vi "Timing Calculator_v2.vi"(8 "Scan settings array":T1[](array[typedef]) {"J-t Illumination conditions" items=["Light only", "Dark only", "Light then dark", "Dark then light"]; "No. of scan rate steps" min=1.0 step=1.0; "Illumination conditions" items=["Light only", "Dark only", "Light then dark", "Dark then light", "Light then dark then light", "Dark then light then dark"]; "Time Constant (s)" items=["0.01s", "0.03s", "0.1s", "0.3s", "1s", "3s"]; "Only repeat for best pixel" items=["only for best pixel", "for best 2 pixels", "for best 3 pixels", "for best 4 pixels", "for best 5 pixels", "for best 6 pixels", "for best 7 pixels", "for all pixels"]; "No. of repeat scans" min=1.0 step=1.0; "EQE best pixel only" items=["only the best pixel", "the best 2 pixel", "the best 3 pixel", "the best 4 pixel", "the best 5 pixel", "the best 6 pixel", "the best 7 pixel", "all pixels"]; "P dep best pixel only" items=["only the best pixel", "the best 2 pixels", "the best 3 pixels", "the best 4 pixels", "the best 5 pixels", "the best 6 pixels", "the best 7 pixels", "all pixels"]; "Max power best pixel only" items=["only the best pixel", "the best 2 pixels", "the best 3 pixels", "the best 4 pixels", "the best 5 pixels", "the best 6 pixels", "the best 7 pixels", "all pixels"]; "J-t best pixel only" items=["only the best pixel", "the best 2 pixels", "the best 3 pixels", "the best 4 pixels", "the best 5 pixels", "the best 6 pixels", "the best 7 pixels", "all pixels"]; "Integration time" items=["Fast", "Normal", "High Accuracy"]; "Stabilisation mode" items=["V", "I"]; "Measurement delay (ms)" min=10.0}, 11 "Measurement queue":T3(array[cluster]) {"Pixel to measure" items=["All", "1", "2", "3", "4", "5", "6", "7", "8"]}) -> (3 "Experiment time (s)":dbl)   [LabVIEW 2011]
uses:
  TypeDefs/Scan settings.ctl
  TypeDefs/Settings Boolean.ctl
panel:
  out "Step time (s)":dbl
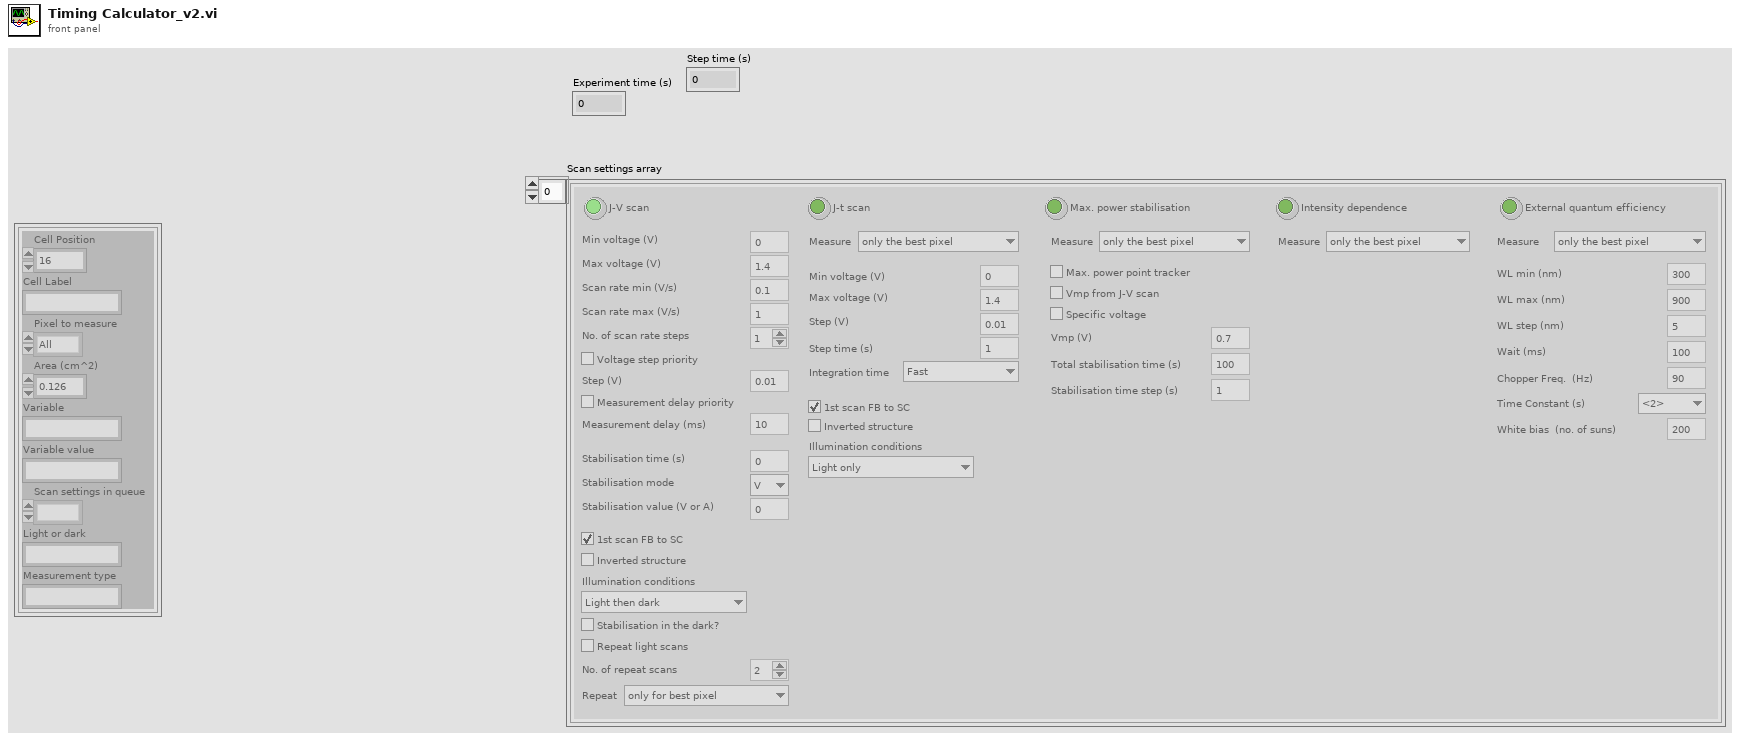
[diagram p1: front panel]
types:
  T1 = typedef "Scan settings.ctl" = cluster{"J-V scan":T2, "J-t scan":bool, "Min voltage (V)":dbl, "Max voltage (V)":dbl, "Step (V)":dbl, "Measurement delay (ms)":dbl, "1st scan FB-SC":bool, "Inverted structure":bool, "Stabilisation time (s)":dbl, "Stabilisation mode":u16, "Stabilisation value (V or A) ":dbl, "Step time (s)":dbl, "Integration time":u16, "Repeat light scans":bool, "Stabilisation in the dark?":bool, "J-t Min (V)":dbl, "J-t Max (V)":dbl, "J-t Step (V)":dbl, "Max. power stabilisation":bool, "J-t 1st scan FB-SC":bool, "J-t Inverted structure":bool, "Max power tracking":bool, "Vmp (V)":dbl, "Total stabilisation time (s)":dbl, "J-t best pixel only":u16, "Max power best pixel only":u16, "Vmp from J-V scan":bool, "Intensity dependence":bool, "P dep best pixel only":u16, "External quantum efficiency":bool, "EQE best pixel only":u16, "WL min (nm)":dbl, "WL max (nm)":dbl, "WL step (nm)":dbl, "Wait (ms)":dbl, "No. of repeat scans":dbl, "Only repeat for best pixel":u16, "Chopper Freq.  (Hz)":dbl, "Time Constant (s)":dbl, "Stabilisation time step (s)":dbl, "Illumination conditions":u16, "Scan rate min (V/s)":dbl, "Scan rate max (V/s)":dbl, "No. of scan rate steps":dbl, "Scan rate voltage step priority":bool, "Scan rate measurement delay priority":bool, "J-t Illumination conditions":u16, "White bias  (no. of suns)":dbl, "Max P stab. Specific voltage":bool}
  T2 = typedef "Settings Boolean.ctl" = bool
  T3 = cluster{"Cell Position":i32, "Cell Label":string, "Pixel to measure":u16, "Area (cm^2)":dbl, "Variable":string, "Variable value":string, "Scan settings in queue":u16, "Light or dark":string, "Measurement type":string}[]
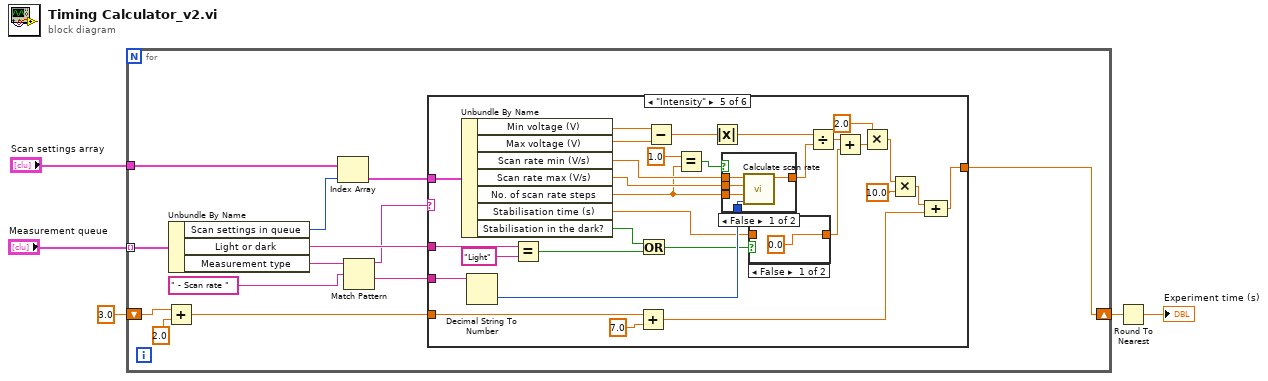
[diagram p0: block diagram]
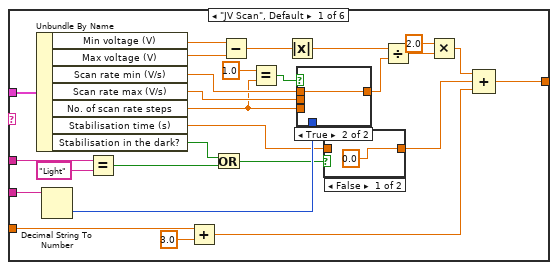
[diagram p2: hidden frame]
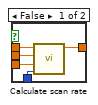
[diagram p4: hidden frame]
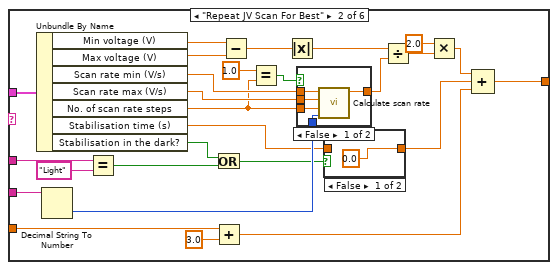
[diagram p5: hidden frame]
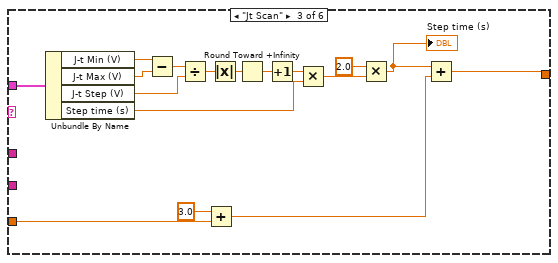
[diagram p8: hidden frame]
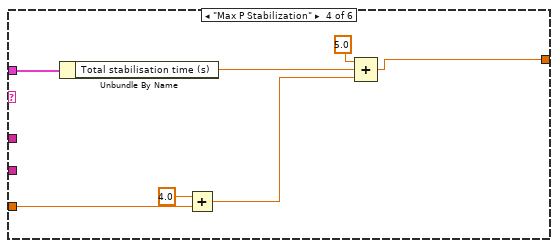
[diagram p9: hidden frame]
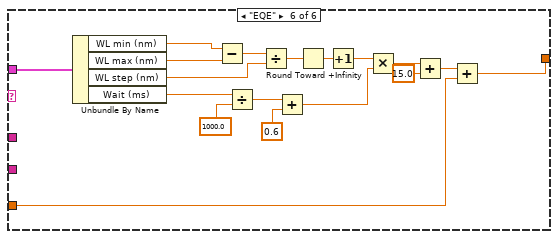
[diagram p12: hidden frame]
diagram:
  n1 = for {
    tunnel: "Measurement queue" -> [w18] mode=indexing
    shift-right: [w6] -> w1
    shift-left: 3.0 -> [w8]
    tunnel: "Scan settings array" -> [w10]
    n2 = Add(x=w8, y=2.0) -> (x+y=w11:dbl)
    n3 = Unbundle By Name(w18) -> ("Scan settings in queue"=w17:u16, "Light or dark"=w12:string, "Measurement type"=w13:string)
    n4 = Index Array(array=w10, index=w17) -> (element=w16:T1)
    n5 = Match Pattern(string=w13, regular expression=" - Scan rate ") -> (before substring=w9:string, after substring=w14:string)  [unwired: 1 in, 2 out]
    n6 = case shown="\"Intensity\"" w9 {
      tunnel: [w43 w78 w97 w109 w126 w151] -> w6
      tunnel: w16 -> [w42 w77 w98 w111 w125 w153]
      tunnel: w14 -> [w40 w75 _ _ w119 _]
      tunnel: w12 -> [w31 w66 _ _ w124 _]
      tunnel: w11 -> [w21 w55 w94 w108 w114 w152]
      frame "JV Scan", Default {
        n7 = Unbundle By Name(w42) -> ("Min voltage (V)"=w45:dbl, "Max voltage (V)"=w44:dbl, "Scan rate min (V/s)"=w37:dbl, "Scan rate max (V/s)"=w38:dbl, "No. of scan rate steps"=w35:dbl, "Stabilisation time (s)"=w29:dbl, "Stabilisation in the dark?"=w28:bool)
        n8 = Decimal String To Number(string=w40) -> (number=w39:i32)  [unwired: 2 in, 1 out]
        n9 = Equal?(x=w31, y="Light") -> (x = y?=w26:bool)
        n10 = Add(x=w21, y=3.0) -> (x+y=w20:dbl)
        n11 = Or(x=w28, y=w26) -> (x .or. y?=w27:bool)
        n12 = Subtract(x=w45, y=w44) -> (x-y=w41:dbl)
        n13 = Equal?(x=1.0 ("y"), y=w35) -> (x = y?=w34:bool)
        n14 = Absolute Value(x=w41) -> (abs(x)=w33:dbl)
        n15 = case shown="True" w34 {
          tunnel: w39 -> [w52 _]
          tunnel: w35 -> [w51 _]
          tunnel: w38 -> [w50 _]
          tunnel: w37 -> [w49 w53]
          tunnel: [w48 w53] -> w32
          frame False {
            n16 = call "Calculate scan rate.vi"("Scan rate number"=w52, "Number of steps"=w51, "Scan rate max (V/s)"=w50, "Scan rate min (V/s)"=w49) -> ("Scan rate"=w48:dbl)  [unwired: 7 in]
          }
          frame True {
          }
        }
        n17 = case shown="False" w27 {
          tunnel: w29 -> [_ w47]
          tunnel: [0.0 ("Stabilisation time (s)") w47] -> w25
          frame False {
          }
          frame True {
          }
        }
        n18 = Divide(x=w33, y=w32) -> (x/y=w24:dbl)
        n19 = Multiply(x=2.0, y=w24) -> (x*y=w22:dbl)
        n20 = Compound Arithmetic op=ADD(w22, w25, w20) -> (w43:dbl)
      }
      frame "Repeat JV Scan For Best" {
        n21 = Unbundle By Name(w77) -> ("Min voltage (V)"=w80:dbl, "Max voltage (V)"=w79:dbl, "Scan rate min (V/s)"=w72:dbl, "Scan rate max (V/s)"=w73:dbl, "No. of scan rate steps"=w70:dbl, "Stabilisation time (s)"=w64:dbl, "Stabilisation in the dark?"=w63:bool)
        n22 = Decimal String To Number(string=w75) -> (number=w74:i32)  [unwired: 2 in, 1 out]
        n23 = Equal?(x=w66, y="Light") -> (x = y?=w61:bool)
        n24 = Or(x=w63, y=w61) -> (x .or. y?=w62:bool)
        n25 = Add(x=w55, y=3.0) -> (x+y=w54:dbl)
        n26 = Subtract(x=w80, y=w79) -> (x-y=w76:dbl)
        n27 = Equal?(x=1.0 ("y"), y=w70) -> (x = y?=w69:bool)
        n28 = Absolute Value(x=w76) -> (abs(x)=w68:dbl)
        n29 = case shown="False" w69 {
          tunnel: w74 -> [w87 _]
          tunnel: w70 -> [w86 _]
          tunnel: w73 -> [w85 _]
          tunnel: w72 -> [w84 w88]
          tunnel: [w83 w88] -> w67
          frame False {
            n30 = call "Calculate scan rate.vi"("Scan rate number"=w87, "Number of steps"=w86, "Scan rate max (V/s)"=w85, "Scan rate min (V/s)"=w84) -> ("Scan rate"=w83:dbl)  [unwired: 7 in]
          }
          frame True {
          }
        }
        n31 = case shown="False" w62 {
          tunnel: w64 -> [_ w82]
          tunnel: [0.0 ("Stabilisation time (s)") w82] -> w60
          frame False {
          }
          frame True {
          }
        }
        n32 = Divide(x=w68, y=w67) -> (x/y=w59:dbl)
        n33 = Multiply(x=2.0, y=w59) -> (x*y=w58:dbl)
        n34 = Compound Arithmetic op=ADD(w58, w60, w54) -> (w78:dbl)
      }
      frame "Jt Scan" {
        n35 = Unbundle By Name(w98) -> ("J-t Min (V)"=w99:dbl, "J-t Max (V)"=w100:dbl, "J-t Step (V)"=w102:dbl, "Step time (s)"=w105:dbl)
        n36 = Subtract(x=w99, y=w100) -> (x-y=w101:dbl)
        n37 = Divide(x=w101, y=w102) -> (x/y=w90:dbl)
        n38 = Add(x=3.0, y=w94) -> (x+y=w93:dbl)
        n39 = Absolute Value(x=w90) -> (abs(x)=w89:dbl)
        n40 = Round Toward +Infinity(x=w89) -> (ceil(x): smallest int >= x=w103:dbl)
        n41 = Increment(x=w103) -> (x+1=w104:dbl)
        n42 = Multiply(x=w104, y=w105) -> (x*y=w96:dbl)
        n43 = Multiply(x=2.0, y=w96) -> (x*y=w91:dbl)
        "Step time (s)" <- w91
        n44 = Add(x=w91, y=w93) -> (x+y=w97:dbl)
      }
      frame "Max P Stabilization" {
        n45 = Unbundle By Name(w111) -> ("Total stabilisation time (s)"=w112:dbl)
        n46 = Add(x=4.0, y=w108) -> (x+y=w106:dbl)
        n47 = Compound Arithmetic op=ADD(5.0 ("value"), w112, w106) -> (w109:dbl)
      }
      frame "Intensity" {
        n48 = Unbundle By Name(w125) -> ("Min voltage (V)"=w142:dbl, "Max voltage (V)"=w141:dbl, "Scan rate min (V/s)"=w137:dbl, "Scan rate max (V/s)"=w138:dbl, "No. of scan rate steps"=w135:dbl, "Stabilisation time (s)"=w130:dbl, "Stabilisation in the dark?"=w129:bool)
        n49 = Decimal String To Number(string=w119) -> (number=w139:i32)  [unwired: 2 in, 1 out]
        n50 = Equal?(x=w124, y="Light") -> (x = y?=w127:bool)
        n51 = Add(x=w114, y=7.0) -> (x+y=w113:dbl)
        n52 = Or(x=w129, y=w127) -> (x .or. y?=w128:bool)
        n53 = Subtract(x=w142, y=w141) -> (x-y=w140:dbl)
        n54 = Equal?(x=1.0 ("y"), y=w135) -> (x = y?=w134:bool)
        n55 = Absolute Value(x=w140) -> (abs(x)=w133:dbl)
        n56 = case shown="False" w134 {
          tunnel: w139 -> [w149 _]
          tunnel: w135 -> [w148 _]
          tunnel: w138 -> [w147 _]
          tunnel: w137 -> [w146 w150]
          tunnel: [w145 w150] -> w132
          frame False {
            n57 = call "Calculate scan rate.vi"("Scan rate number"=w149, "Number of steps"=w148, "Scan rate max (V/s)"=w147, "Scan rate min (V/s)"=w146) -> ("Scan rate"=w145:dbl)  [unwired: 7 in]
          }
          frame True {
          }
        }
        n58 = case shown="False" w128 {
          tunnel: w130 -> [_ w144]
          tunnel: [0.0 ("Stabilisation time (s)") w144] -> w121
          frame False {
          }
          frame True {
          }
        }
        n59 = Divide(x=w133, y=w132) -> (x/y=w122:dbl)
        n60 = Add(x=w122, y=w121) -> (x+y=w117:dbl)
        n61 = Multiply(x=2.0, y=w117) -> (x*y=w118:dbl)
        n62 = Multiply(x=w118, y=10.0) -> (x*y=w120:dbl)
        n63 = Compound Arithmetic op=ADD(w120, w113) -> (w126:dbl)
      }
      frame "EQE" {
        n64 = Unbundle By Name(w153) -> ("WL min (nm)"=w158:dbl, "WL max (nm)"=w159:dbl, "WL step (nm)"=w160:dbl, "Wait (ms)"=w162:dbl)
        n65 = Subtract(x=w158, y=w159) -> (x-y=w154:dbl)
        n66 = Divide(x=w162, y=1000.0) -> (x/y=w164:dbl)
        n67 = Divide(x=w154, y=w160) -> (x/y=w155:dbl)
        n68 = Add(x=w164, y=0.6) -> (x+y=w165:dbl)
        n69 = Round Toward +Infinity(x=w155) -> (ceil(x): smallest int >= x=w156:dbl)
        n70 = Increment(x=w156) -> (x+1=w157:dbl)
        n71 = Multiply(x=w157, y=w165) -> (x*y=w166:dbl)
        n72 = Add(x=w166, y=15.0) -> (x+y=w168:dbl)
        n73 = Add(x=w168, y=w152) -> (x+y=w151:dbl)
      }
    }
  }
  n74 = Round To Nearest(number=w1) -> (nearest integer value=→"Experiment time (s)":dbl)
